vi "Init_Images.vi"() -> (3 "Images":T1)   [LabVIEW 2012]
uses:
  Image Cluster.ctl
  <vilib>/vision/Image Controls.llb/IMAQ Image.ctl
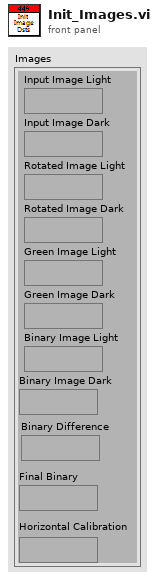
[diagram p1: front panel]
types:
  T1 = typedef "Image Cluster.ctl" = cluster{"Input Image Light":T2, "Input Image Dark":T2, "Rotated Image Light":T2, "Rotated Image Dark":T2, "Green Image Light":T2, "Green Image Dark":T2, "Binary Image Light":T2, "Binary Difference":T2, "Binary Image Dark":T2, "Final Binary":T2, "Horizontal Calibration":T2}
  T2 = typedef "IMAQ Image.ctl" = refnum<image>
  T3 = typedef "Image Type" = u32
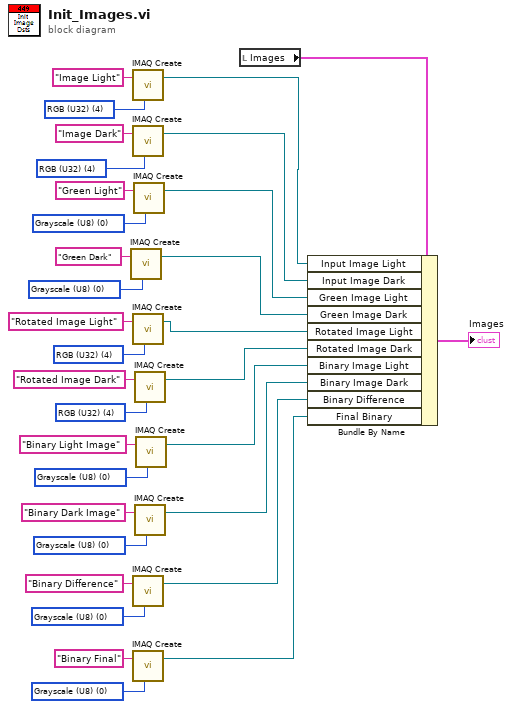
[diagram p0: block diagram]
diagram:
  w3 = T3 0 items=["Grayscale (U8)", "Grayscale (I16)", "Grayscale (SGL)", "Complex (CSG)", "RGB (U32)", "HSL (U32)", "RGB (U64)", "Grayscale (U16)"] ("Image Type")
  w6 = T3 0 items=["Grayscale (U8)", "Grayscale (I16)", "Grayscale (SGL)", "Complex (CSG)", "RGB (U32)", "HSL (U32)", "RGB (U64)", "Grayscale (U16)"] ("Image Type")
  w8 = T3 4 items=["Grayscale (U8)", "Grayscale (I16)", "Grayscale (SGL)", "Complex (CSG)", "RGB (U32)", "HSL (U32)", "RGB (U64)", "Grayscale (U16)"] ("Image Type")
  w9 = T3 4 items=["Grayscale (U8)", "Grayscale (I16)", "Grayscale (SGL)", "Complex (CSG)", "RGB (U32)", "HSL (U32)", "RGB (U64)", "Grayscale (U16)"] ("Image Type")
  w11 = T3 0 items=["Grayscale (U8)", "Grayscale (I16)", "Grayscale (SGL)", "Complex (CSG)", "RGB (U32)", "HSL (U32)", "RGB (U64)", "Grayscale (U16)"] ("Image Type")
  w14 = T3 0 items=["Grayscale (U8)", "Grayscale (I16)", "Grayscale (SGL)", "Complex (CSG)", "RGB (U32)", "HSL (U32)", "RGB (U64)", "Grayscale (U16)"] ("Image Type")
  w26 = T3 0 items=["Grayscale (U8)", "Grayscale (I16)", "Grayscale (SGL)", "Complex (CSG)", "RGB (U32)", "HSL (U32)", "RGB (U64)", "Grayscale (U16)"] ("Image Type")
  w27 = T3 0 items=["Grayscale (U8)", "Grayscale (I16)", "Grayscale (SGL)", "Complex (CSG)", "RGB (U32)", "HSL (U32)", "RGB (U64)", "Grayscale (U16)"] ("Image Type")
  w29 = T3 4 items=["Grayscale (U8)", "Grayscale (I16)", "Grayscale (SGL)", "Complex (CSG)", "RGB (U32)", "HSL (U32)", "RGB (U64)", "Grayscale (U16)"] ("Image Type")
  w31 = T3 4 items=["Grayscale (U8)", "Grayscale (I16)", "Grayscale (SGL)", "Complex (CSG)", "RGB (U32)", "HSL (U32)", "RGB (U64)", "Grayscale (U16)"] ("Image Type")
  n1 = call "IMAQ Create"("Image Name"="Green Dark", "Image Type"=w26) -> ("New Image"=w17:T2)  [unwired: 3 in, 1 out]
  n2 = call "IMAQ Create"("Image Name"="Image Light", "Image Type"=w8) -> ("New Image"=w20:T2)  [unwired: 3 in, 1 out]
  n3 = call "IMAQ Create"("Image Name"="Image Dark", "Image Type"=w9) -> ("New Image"=w19:T2)  [unwired: 3 in, 1 out]
  n4 = call "IMAQ Create"("Image Name"="Rotated Image Light", "Image Type"=w29) -> ("New Image"=w16:T2)  [unwired: 3 in, 1 out]
  n5 = call "IMAQ Create"("Image Name"="Binary Difference", "Image Type"=w11) -> ("New Image"=w5:T2)  [unwired: 3 in, 1 out]
  n6 = call "IMAQ Create"("Image Name"="Binary Final", "Image Type"=w3) -> ("New Image"=w1:T2)  [unwired: 3 in, 1 out]
  n7 = call "IMAQ Create"("Image Name"="Green Light", "Image Type"=w27) -> ("New Image"=w18:T2)  [unwired: 3 in, 1 out]
  n8 = call "IMAQ Create"("Image Name"="Rotated Image Dark", "Image Type"=w31) -> ("New Image"=w15:T2)  [unwired: 3 in, 1 out]
  n9 = call "IMAQ Create"("Image Name"="Binary Dark Image", "Image Type"=w6) -> ("New Image"=w4:T2)  [unwired: 3 in, 1 out]
  n10 = call "IMAQ Create"("Image Name"="Binary Light Image", "Image Type"=w14) -> ("New Image"=w10:T2)  [unwired: 3 in, 1 out]
  n11 = local read "Images"() -> (w22:T1)
  n12 = Bundle By Name(cluster=w22, "Input Image Light"=w20, "Input Image Dark"=w19, "Green Image Light"=w18, "Green Image Dark"=w17, "Rotated Image Light"=w16, "Rotated Image Dark"=w15, "Binary Image Light"=w10, "Binary Image Dark"=w4, "Binary Difference"=w5, "Final Binary"=w1) -> (→"Images":T1)
